vi "CRYCal Intensity.vi"(6 "map selector":T2(ring)=enum."rainbow", 8 "window info":cluster{"type":T1, "length":i32}={"type"=1, "length"=64} {"type" items=["Rectangle"=0, "Hanning"=1, "Hamming"=2, "Blackman-Harris"=3, "Exact Blackman"=4, "Blackman"=5, "Flat Top"=6, "4 Term B-Harris "=7, "7 Term B-Harris"=8, "Low Sidelobe"=9, "Blackman Nuttall"=11, "Triangle"=30, "Bartlett-Hanning"=31, "Bohman"=32, "Parzen"=33, "Welch"=34, "Kaiser"=60, "Dolph-Chebyshev"=61, "Gaussian"=62]}, 9 "time-freq sampling info":cluster{"time steps":i32, "frequency bins":i32}={"time steps"=512, "frequency bins"=1024}, 10 "Fs":dbl, 11 "Y":dbl[](array[numeric])) -> (3 "STFT Spectrum":dbl[][](array[numeric]))   [LabVIEW 2013]
uses:
  <vilib>/Analysis/4window.llb/windowTd.ctl
  <vilib>/gmath/NI_Gmath.lvlib
  <vilib>/Analysis/NI_AALPro.lvlib
panel:
  out "STFT Spectrogram":dbl[][](graph)
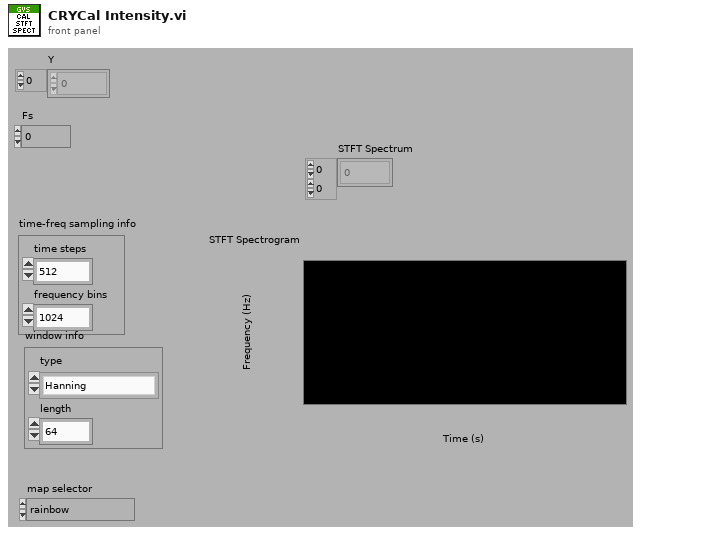
[diagram p1: front panel]
types:
  T1 = typedef "NI_AALPro.lvlib/windowTd.ctl" = u32
  T2 = enum16{"fire", "rainbow", "grey", "inverse grey", "ice", "original"}
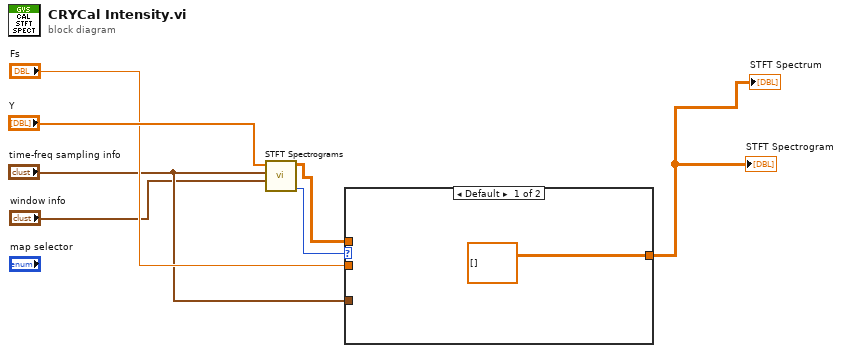
[diagram p0: block diagram]
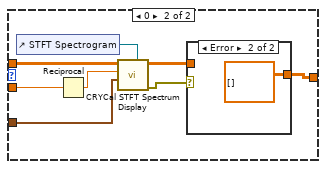
[diagram p2: hidden frame]
diagram:
  n1 = call <vilib>:"STFT Spectrograms.vi"("window info"="window info", "time-freq sampling info"="time-freq sampling info", "X"="Y") -> ("error"=w6:i32, "STFT Spectrogram {X}"=w4:dbl[][])  [unwired: 3 in, 4 out]
  n2 = case shown="Default" w6 {
    tunnel: [dbl[][] [] ("STFT Spectrogram Out") w14] -> w5
    tunnel: w4 -> [_ w16]
    tunnel: "Fs" -> [_ w11]
    tunnel: "time-freq sampling info" -> [_ w9]
    frame Default {
    }
    frame 0 {
      n3 = control-ref of="STFT Spectrogram"() -> (w12:refnum<vi>)
      n4 = Reciprocal(x=w11) -> (1/x=w10:dbl)
      n5 = call "CRYCal STFT Spectrum Display.vi"("Intensity Graph"=w12, "time-freq sampling info"=w9, "dt"=w10, "STFT Spectrogram In"=w16) -> ("error out"=w15:errorcluster, "STFT Spectrogram Out"=w13:dbl[][])  [unwired: 3 in, 3 out]
      n6 = case shown="Error" w15 {
        tunnel: [w17 dbl[][] [] ("STFT Spectrogram Out")] -> w14
        tunnel: w13 -> [w17 _]
        frame No Error {
        }
        frame Error {
        }
      }
    }
  }
  "STFT Spectrogram" <- w5
  "STFT Spectrum" <- w5
